vi "KEI_Voltage.vi"(3 "error in":errorcluster, 4 "Language":T1, 5 "voltageList":string, 6 "GPIB":refnum<visa-resource-name>="GPIB0::16::INSTR") -> (0 "error out":errorcluster, 1 "Message":string, 2 "voltage":dbl[](array[numeric]))   [LabVIEW 2015]
doc: "记录端电压\nunIndex：-1断路器未安装，端电压为-1"
uses:
  CustomControl/Lang_Control.ctl
  <instrlib>/Keithley 27XX/Public/Data/Read Multiple Direct.vi
  <instrlib>/Keithley 27XX/Keithley 27XX.lvlib
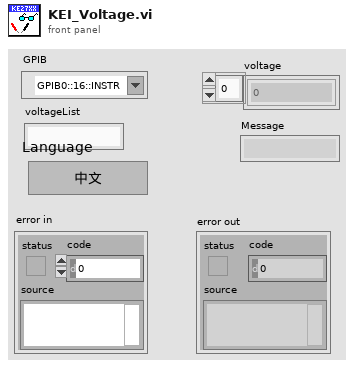
[diagram p1: front panel]
types:
  T1 = typedef "Lang_Control.ctl" = enum16{"中文", "English"}
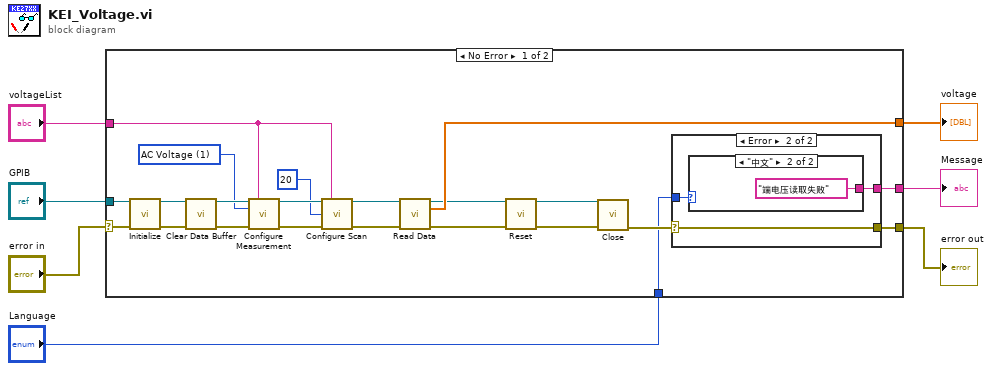
[diagram p0: block diagram]
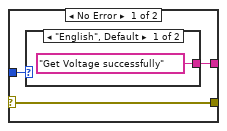
[diagram p2: hidden frame]
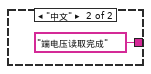
[diagram p3: hidden frame]
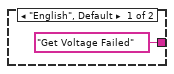
[diagram p4: hidden frame]
diagram:
  n1 = case shown="No Error" "error in" {
    selector: "error in" -> [w16 w40]
    tunnel: "voltageList" -> [w21 _]
    tunnel: [w20 _] -> w6
    tunnel: "GPIB" -> [w17 _]
    tunnel: [w14 w40] -> w3
    tunnel: [w13 _] -> w2
    tunnel: "Language" -> [w12 _]
    frame No Error {
      w27 = u16 1 items=["DC Voltage", "AC Voltage", "DC Current", "AC Current", "Resistance", "Four-Wire Resistance", "Temperature", "Frequency", "Period", "Continuity"] ("Function (0: DC Voltage)")
      n2 = call <instrlib>:"Initialize.vi"("VISA resource name"=w17, "error in (no error)"=w16) -> ("VISA resource name out"=w19:refnum<visa-resource-name>, "error out"=w18:errorcluster)  [unwired: 12 in]
      n3 = call <instrlib>:"Clear Data Buffer.vi"("VISA resource name"=w19, "error in (no error)"=w18) -> ("VISA resource name out"=w29:refnum<visa-resource-name>, "error out"=w28:errorcluster)  [unwired: 12 in]
      n4 = call <instrlib>:"Configure Measurement.vi"("VISA resource name"=w29, "Scan List (Empty)"=w21, "Function (0: DC Voltage)"=w27, "error in (no error)"=w28) -> ("VISA resource name out"=w26:refnum<visa-resource-name>, "error out"=w25:errorcluster)  [unwired: 10 in]
      n5 = call <instrlib>:"Configure Scan.vi"("VISA resource name"=w26, "Channel List (101:110)"=w21, "Sample Count (100)"=20, "error in (no error)"=w25) -> ("VISA resource name out"=w23:refnum<visa-resource-name>, "error out"=w22:errorcluster)  [unwired: 10 in]
      n6 = call-poly <instrlib>:"Read Data.vi"("VISA resource name"=w23, "error in (no error)"=w22) -> ("VISA resource name out"=w11:refnum<visa-resource-name>, "Measurement Data"=w20:dbl[], "error out"=w9:errorcluster)  [unwired: 8 in, 3 out]
      n7 = call <instrlib>:"Reset.vi"("VISA resource name"=w11, "error in (no error)"=w9) -> ("VISA resource name out"=w10:refnum<visa-resource-name>, "error out"=w8:errorcluster)  [unwired: 12 in]
      n8 = call <instrlib>:"Close.vi"("VISA resource name"=w10, "error in (no error)"=w8) -> ("error out"=w15:errorcluster)  [unwired: 13 in]
      n9 = case shown="Error" w15 {
        selector: w15 -> [w32 w37]
        tunnel: [w32 w37] -> w14
        tunnel: [w31 w36] -> w13
        tunnel: w12 -> [w30 w35]
        frame No Error {
          n10 = case shown="\"English\", Default" w30 {
            tunnel: ["Get Voltage successfully" ("error source (\" \")") "端电压读取完成" ("error source (\" \")")] -> w31
            frame "English", Default {
            }
            frame "中文" {
            }
          }
        }
        frame Error {
          n11 = case shown="\"中文\"" w35 {
            tunnel: ["Get Voltage Failed" ("error source (\" \")") "端电压读取失败" ("error source (\" \")")] -> w36
            frame "English", Default {
            }
            frame "中文" {
            }
          }
        }
      }
    }
    frame Error {
    }
  }
  "voltage" <- w6
  "error out" <- w3
  "Message" <- w2
